vi "DllFxpAddSub_BoolArray.vi"(6 "cin/nbin":bool, 8 "load":bool=TRUE, 9 "is sub":bool, 10 "y":bool[](array[boolean])=[FALSE, FALSE, FALSE, FALSE, FALSE, FALSE, FALSE, FALSE, FALSE, FALSE, FALSE, FALSE, FALSE, FALSE, FALSE, FALSE], 11 "x":bool[](array[boolean])=[FALSE, FALSE, FALSE, FALSE, FALSE, FALSE, FALSE, FALSE, FALSE, FALSE, FALSE, FALSE, FALSE, FALSE, FALSE, FALSE]) -> (2 "cout/nbout/overflow":bool, 3 "s":bool[](array[boolean]))   [LabVIEW 2017]
uses:
  <vilib>/rvi/FXPMathLib/sim/FxpSim.dll
panel:
  # "First element is LSB"
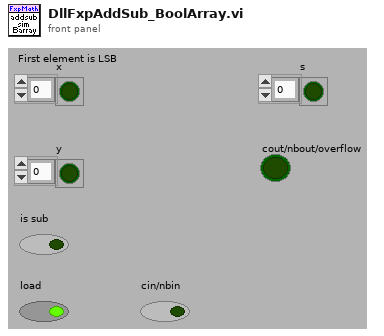
[diagram p1: front panel]
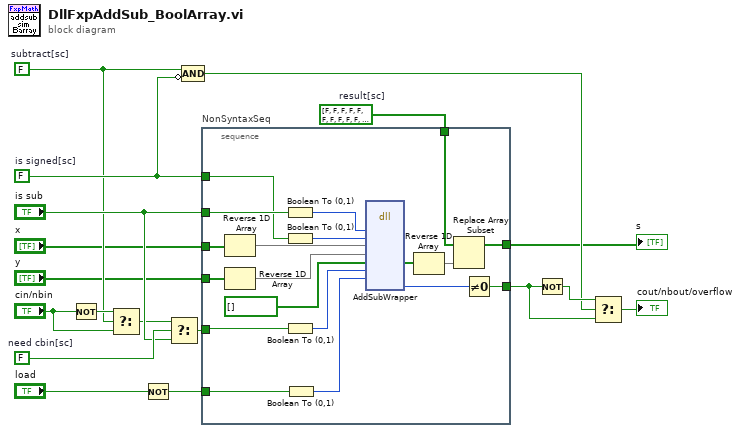
[diagram p0: block diagram]
diagram:
  w1 = bool[] [FALSE, FALSE, FALSE, FALSE, FALSE, FALSE, FALSE, FALSE, FALSE, FALSE, FALSE, FALSE, FALSE, FALSE, FALSE, FALSE]  # result[sc]
  w6 = FALSE  # subtract[sc]
  w7 = FALSE  # is signed[sc]
  w18 = FALSE  # need cbin[sc]
  n1 = Not(x="cin/nbin") -> (.not. x?=w12:bool)
  n2 = Select(t=w12, s=w6, f="cin/nbin") -> (s? t:f=w14:bool)
  n3 = Not(x="load") -> (.not. x?=w13:bool)
  n4 = Select(t=w14, s=w18, f="is sub") -> (s? t:f=w16:bool)
  n5 = Compound Arithmetic op=AND(w6, invert w7) -> (w5:bool)
  n6 = stacked-sequence "NonSyntaxSeq" {
    tunnel: [w37] -> w9
    tunnel: "is sub" -> [w36]
    tunnel: "x" -> [w22]
    tunnel: "y" -> [w20]
    tunnel: w16 -> [w33]
    tunnel: w13 -> [w32]
    tunnel: w7 -> [w31]
    tunnel: [w25] -> w2
    tunnel: w1 -> [w26]
    frame #0 {
      n7 = Reverse 1D Array(array=w22) -> (reversed array=w21:bool[])
      n8 = Reverse 1D Array(array=w20) -> (reversed array=w19:bool[])
      n9 = Boolean To (0,1)(Boolean=w36) -> (0, 1=w35:i16)
      n10 = Boolean To (0,1)(Boolean=w31) -> (0, 1=w34:i16)
      n11 = Boolean To (0,1)(Boolean=w33) -> (0, 1=w30:i16)
      n12 = Boolean To (0,1)(Boolean=w32) -> (0, 1=w28:i16)
      n13 = dll-call lib="e:/penguin/lvdist/win32/export/17.0/17.0.1f1/dist/vi.lib/rvi/FXPMathLib/sim/FxpSim.dll" fn="AddSubWrapper"("isSub"=w35, "isSigned"=w34, "xH"=w21, "yH"=w19, "zH"=bool[] [] ("xH"), "CinOrNBin"=w30, "notLoad"=w28) -> ("zH"=w24:bool[], "CoutOrNBoutOrOvfl"=w29:u8)  [unwired: 3 in, 10 out]
      n14 = Reverse 1D Array(array=w24) -> (reversed array=w23:bool[])
      n15 = Replace Array Subset(array=w26, new element=w23) -> (w25:bool[])  [unwired: 1 in]
      n16 = Not Equal To 0?(x=w29) -> (x != 0?=w37:bool)
    }
  }
  "s" <- w2
  n17 = Not(x=w9) -> (.not. x?=w10:bool)
  n18 = Select(t=w10, s=w5, f=w9) -> (s? t:f=→"cout/nbout/overflow":bool)
